vi "Rogers_GCode.vi"(7 "cmd amd State":cluster{"Command":string, "End State":dbl[]}[](array[cluster]), 8 "Setup":T1={"Scaling (pixels/mm)"=1.0, "Tool Diameter (inch)"=0.25, "Origin location"={"x (mm)"=10, "y (mm)"=300}, "Wood dim"={"width (inch)"=10.0, "height (inch)"=300.0}}, 9 "SubCut":cluster{dbl, dbl}(slide)={0.0, 46.55172413793103} scale=0.0..1.0, 10 "Commands in":string[](array[string])) -> (1 "Cut":picture, 2 "Commands":string[](array[string]), 3 "Bounds":T2 {"Z Max" format="%#.1f"; "Z Min" format="%#.1f"; "Y Max" format="%#.1f"; "Y Min" format="%#.1f"; "X Max" format="%#.1f"; "X Min" format="%#.1f"})   [LabVIEW 2024]
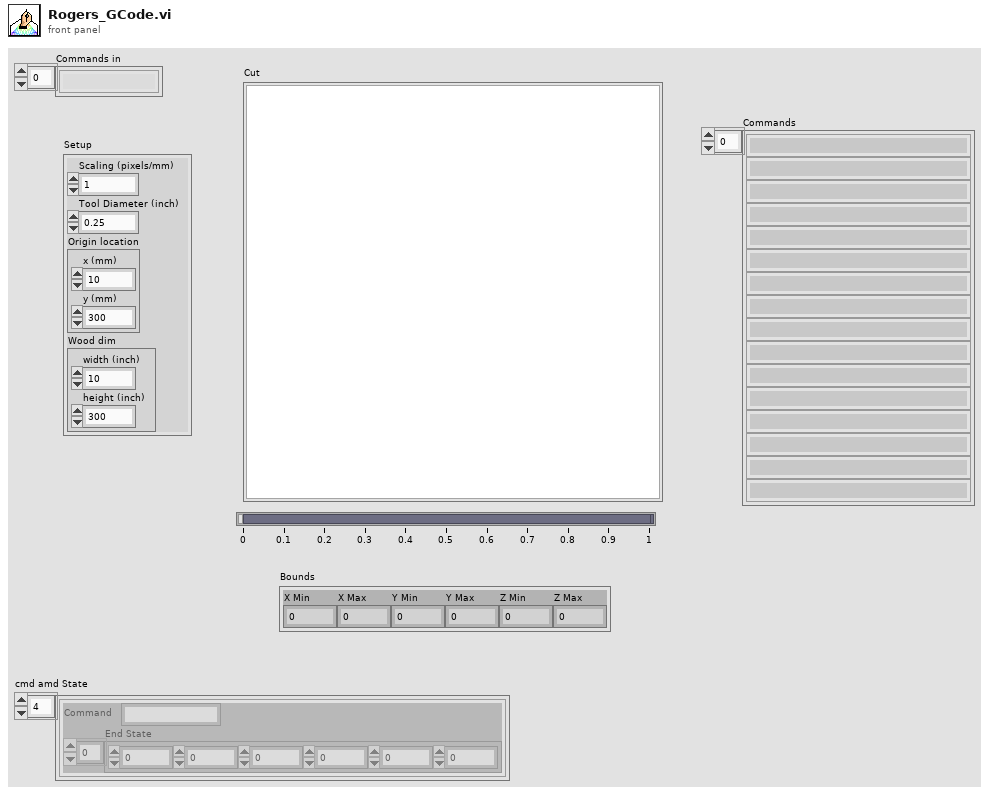
[diagram p1: front panel]
types:
  T1 = cluster{"Scaling (pixels/mm)":dbl, "Tool Diameter (inch)":dbl, "Origin location":cluster{"x (mm)":i16, "y (mm)":i16}, "Wood dim":cluster{"width (inch)":dbl, "height (inch)":dbl}}
  T2 = cluster{"X Min":dbl, "X Max":dbl, "Y Min":dbl, "Y Max":dbl, "Z Min":dbl, "Z Max":dbl}
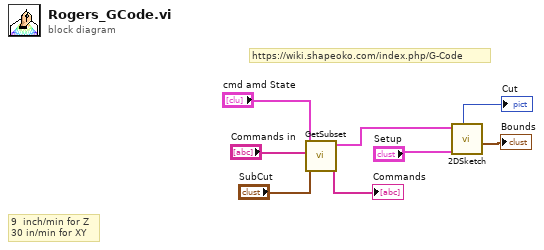
[diagram p0: block diagram]
diagram:
  # "9  inch/min for Z\n30 in/min for XY"
  # "https://wiki.shapeoko.com/index.php/G-Code"
  n1 = call "GetSubset.vi"("SubCut"="SubCut", "Commands in"="Commands in", "cmd amd State"="cmd amd State") -> ("Commands out"=→"Commands":string[], "cmd amd State out"=w4:cluster{"Command":string, "End State":dbl[]}[])  [unwired: 7 in]
  n2 = call "2DSketch.vi"("Setup"="Setup", "cmd amd State"=w4) -> ("Bounds"=→"Bounds":T2, "Cut"=→"Cut":picture)  [unwired: 8 in]
